vi "Refresh Feed (By URI).vi"(8 "error in (no error)":errorcluster, 11 "feed URI in":string) -> (0 "error out":errorcluster, 3 "feed URI out":string)   [LabVIEW 2014, in "NIPM_API.lvlib"]
doc: "Refreshes NI Package Manager with data from the specified feed. \n\nFeed URI - This input must refer to a registered feed. This input cannot be an empty string.\nNote: Feed names are case-sensitive."
uses:
  NIPM_API.lvlib
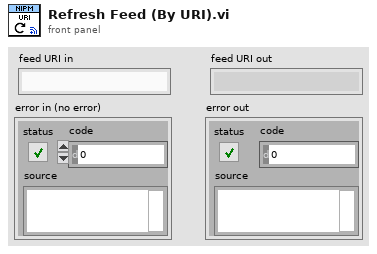
[diagram p1: front panel]
types:
  T1 = typedef "NIPM_API.lvlib/feed.ctl" = cluster{"Name":string, "URI":string}
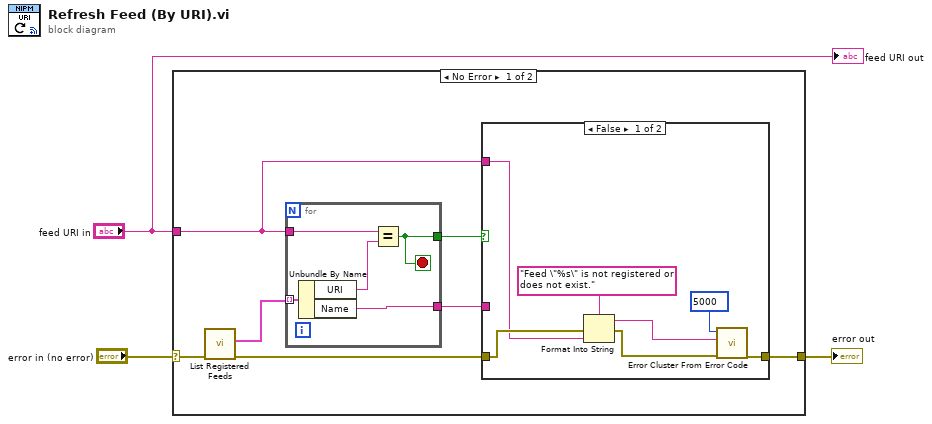
[diagram p0: block diagram]
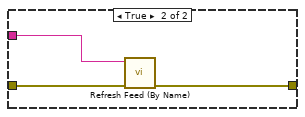
[diagram p2: hidden frame]
diagram:
  n1 = case shown="No Error" "error in (no error)" {
    selector: "error in (no error)" -> [w4 w26]
    tunnel: [w10 w26] -> w3
    tunnel: "feed URI in" -> [w7 _]
    frame No Error {
      n2 = call "List Registered Feeds.vi"("error in"=w4) -> ("error out"=w8:errorcluster, "registered feeds"=w5:T1[])  [unwired: 9 in]
      n3 = for {
        tunnel: w7 -> [w24]
        tunnel: w5 -> [w25] mode=indexing
        tunnel: [w22] -> w6
        tunnel: [w21] -> w9
        stop <- w22 stop-if-true
        n4 = Unbundle By Name(w25) -> ("URI"=w23:string, "Name"=w21:string)
        n5 = Equal?(x=w24, y=w23) -> (x = y?=w22:bool)
      }
      n6 = case shown="False" w6 {
        tunnel: w8 -> [w13 w20]
        tunnel: [w12 w19] -> w10
        tunnel: w7 -> [w11 _]
        tunnel: w9 -> [_ w18]
        frame False {
          n7 = Format Into String(format string="Feed \"%s\" is not registered or does not exist.", error in=w13, w11) -> (resulting string=w14:string, error out=w15:errorcluster)  [unwired: 1 in]
          n8 = call <vilib>:"Error Cluster From Error Code.vi"("error in (no error)"=w15, "error message (\"\")"=w14, "error code (0)"=5000) -> ("error out"=w12:errorcluster)  [unwired: 6 in]
        }
        frame True {
          n9 = call "Refresh Feed (By Name).vi"("error in"=w20, "feed name in"=w18) -> ("error out"=w19:errorcluster)  [unwired: 8 in, 1 out]
        }
      }
    }
    frame Error {
    }
  }
  "error out" <- w3
  "feed URI out" <- "feed URI in"
